vi "Grid_FixOrder.vi"() -> ()   [LabVIEW 2014]
uses:
  <userlib>/Nanonis Prog Interface V5/Nanonis Prog Interface.lvlib
panel:
  in  "Binary Spectroscopy File":path
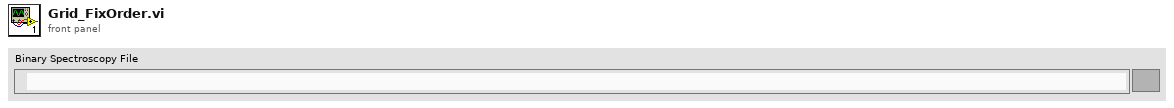
[diagram p1: front panel]
types:
  T1 = typedef "Nanonis Prog Interface.lvlib/Binary_SpectroscopyFile-Config.ctl" = cluster{"Num Par":i32, "Exp size":i32, "Points":i32, "Grid Dim X":i32, "Grid Dim Y":i32, "Header size":i32, "Channels":string[], "Parameters":string[], "Sweep Signal":string, "Grid":cluster{"center X (m)":sgl, "center Y (m)":sgl, "width (m)":sgl, "height (m)":sgl, "angle (deg)":sgl}}
  T2 = cluster{"center X (m)":sgl, "center Y (m)":sgl, "width (m)":sgl, "height (m)":sgl, "angle (deg)":sgl}
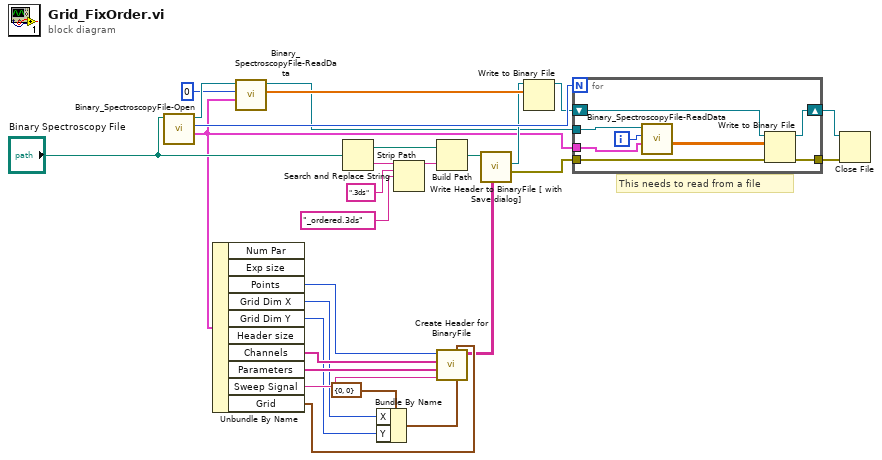
[diagram p0: block diagram]
diagram:
  # "This needs to read from a file"
  n1 = call <userlib>:"Binary_SpectroscopyFile-Open.vi"("Binary Spectroscopy File"="Binary Spectroscopy File") -> ("Config"=w1:T1, "Number of Experiments"=w27:i32, "File ref"=w4:refnum<file>)  [unwired: 6 in, 2 out]
  n2 = Unbundle By Name(w1) -> ("Points"=w12:i32, "Grid Dim X"=w14:i32, "Grid Dim Y"=w13:i32, "Channels"=w18:string[], "Parameters"=w19:string[], "Sweep Signal"=w20:string, "Grid"=w17:T2)  [unwired: 3 out]
  n3 = call <userlib>:"Binary_SpectroscopyFile-ReadData.vi"("Config"=w1, "Experiment to read (Index)"=0, "File ref In"=w4) -> ("Parameter values"=w7:sgl[], "File ref Out"=w3:refnum<file>)  [unwired: 5 in, 2 out]
  n4 = Strip Path(path="Binary Spectroscopy File") -> (stripped path=w28:path, name=w24:string)
  n5 = Bundle By Name(cluster=cluster{"X":i32, "Y":i32} {"X"=0, "Y"=0} ("Grid points"), "X"=w14, "Y"=w13) -> (w15:cluster{"X":i32, "Y":i32})
  n6 = Search and Replace String(input string=w24, search string=".3ds", replace string="_ordered.3ds" ("string")) -> (result string=w21:string)  [unwired: 5 in, 3 out]
  n7 = Build Path(base path=w28, name or relative path=w21) -> (appended path=w10:path)
  n8 = call <userlib>:"Create Header for BinaryFile.vi"("Grid points"=w15, "Grid param"=w17, "Sweep signal"=w20, "Parameters"=w19, "Channels"=w18, "Points per sweep"=w12) -> ("Header (fixed attributes)"=w11:string[][])  [unwired: 5 in]
  n9 = call <userlib>:"Write Header to BinaryFile [ with Save dialog].vi"("Fixed Attributes"=w11, "Filename"=w10) -> ("Error out"=w8:errorcluster, "File ref"=w6:refnum<file>)  [unwired: 6 in, 2 out]
  n10 = Write to Binary File(file (use dialog)=w6, data=w7) -> (refnum out=w5:refnum<file>)  [unwired: 4 in, 2 out]
  n11 = for {
    N: w27 -> [_]
    tunnel: w3 -> [w36]
    tunnel: w1 -> [w35]
    tunnel: w8 -> [w34]
    shift-right: [w31] -> w26
    shift-left: w5 -> [w33]
    tunnel: [w29] -> w25
    i -> [w30]
    n12 = call <userlib>:"Binary_SpectroscopyFile-ReadData.vi"("Config"=w35, "Experiment to read (Index)"=w30, "File ref In"=w36) -> ("data"=w32:sgl[][])  [unwired: 5 in, 3 out]
    n13 = Write to Binary File(file (use dialog)=w33, data=w32, error in=w34) -> (refnum out=w31:refnum<file>, error out=w29:errorcluster)  [unwired: 3 in, 1 out]
  }
  n14 = Close File(refnum=w26, error in=w25) -> ()  [unwired: 2 out]
